vi "registrationEtlZDynamic.vi"() -> ()   [LabVIEW 2017]
uses:
  globalDevices.vi
  globalUtilities.vi
panel:
  in  "stop":bool
  out "z-profile":cluster{dbl[], dbl[]}[](graph)
  in  "newVolume":bool
  # "1. Check that the peak does not move. This will check that\nyou have the right etlLatencyShift\n2. Check that when you set a value you get the correct position\nin the other lens' space."
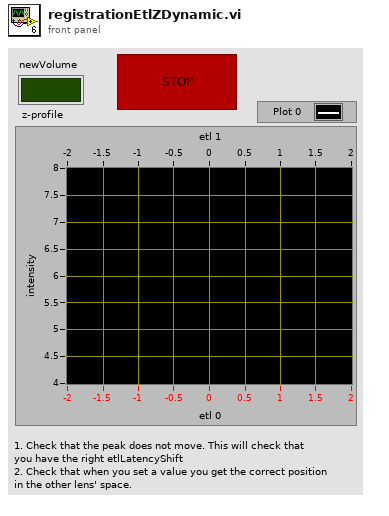
[diagram p1: front panel]
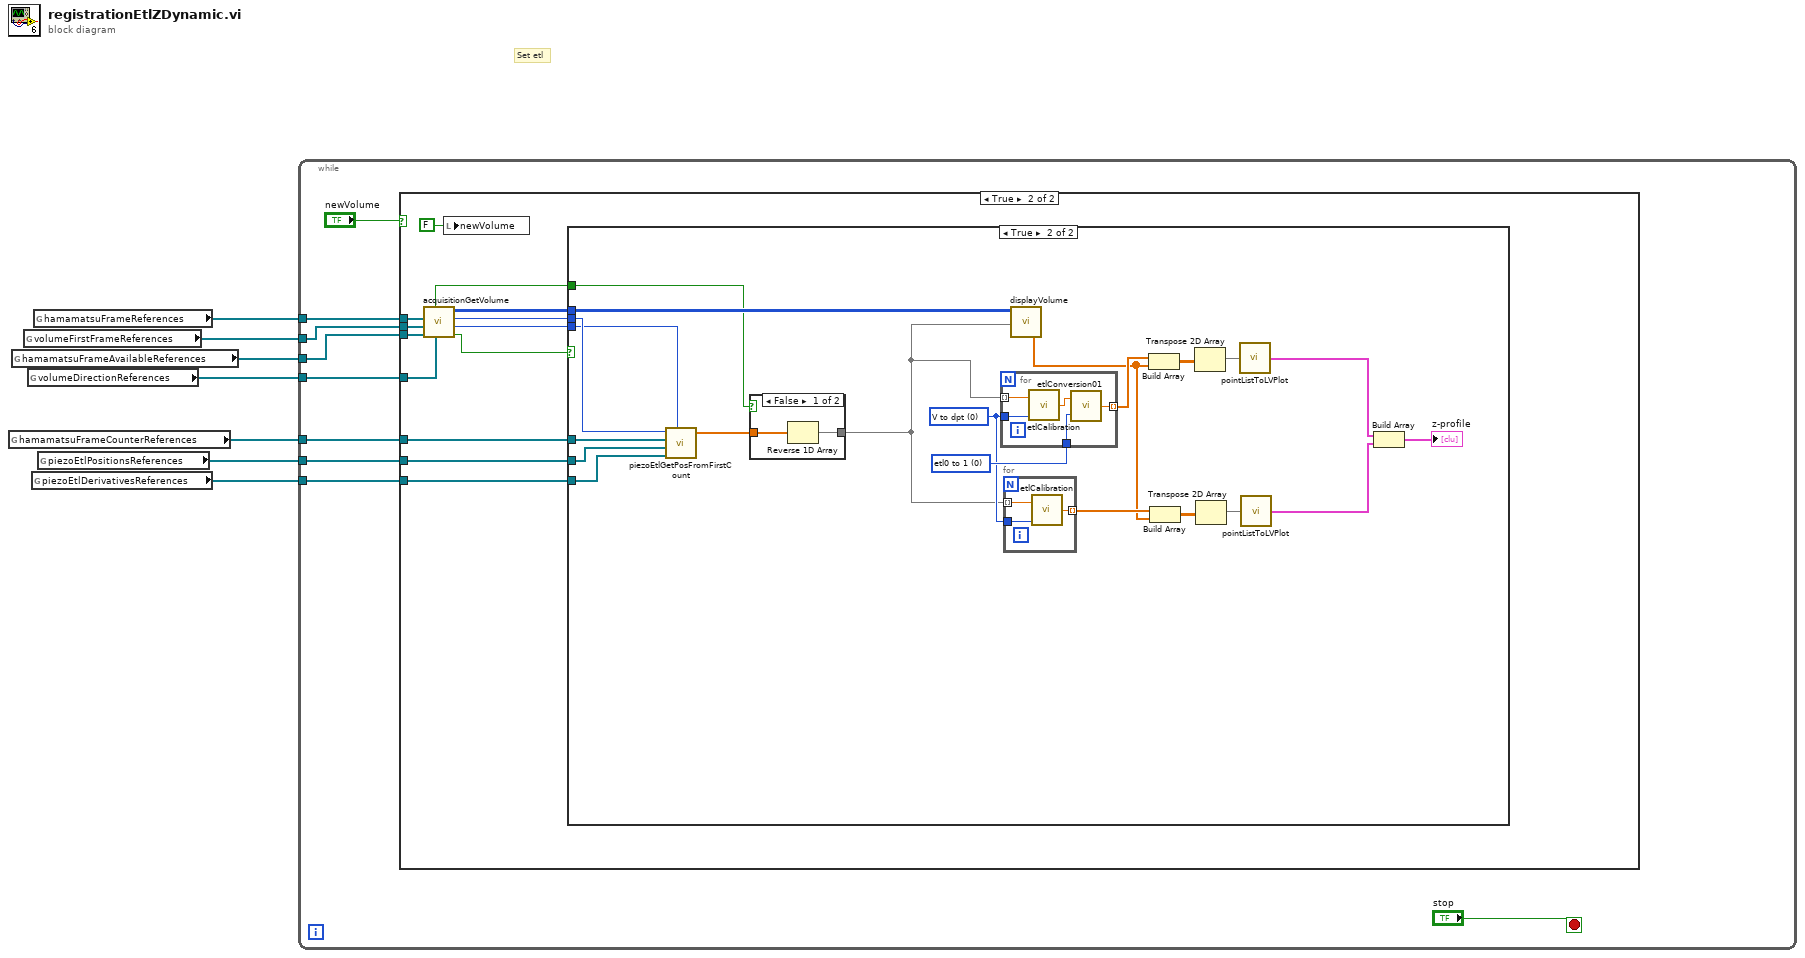
[diagram p0: block diagram]
diagram:
  # "Set etl"
  n1 = global read "globalDevices.vi" "hamamatsuFrameCounterReferences"() -> (w3:refnum<data-value>[])
  n2 = global read "globalDevices.vi" "hamamatsuFrameAvailableReferences"() -> (w5:refnum<data-value>[])
  n3 = global read "globalUtilities.vi" "volumeFirstFrameReferences"() -> (w6:refnum<data-value>[])
  n4 = global read "globalUtilities.vi" "volumeDirectionReferences"() -> (w4:refnum<data-value>[])
  n5 = global read "globalDevices.vi" "piezoEtlDerivativesReferences"() -> (w1:refnum<data-value>[])
  n6 = global read "globalDevices.vi" "hamamatsuFrameReferences"() -> (w7:refnum<data-value>[])
  n7 = global read "globalDevices.vi" "piezoEtlPositionsReferences"() -> (w2:refnum<data-value>[])
  n8 = while {
    tunnel: w7 -> [w16]
    tunnel: w6 -> [w15]
    tunnel: w5 -> [w14]
    tunnel: w4 -> [w13]
    tunnel: w3 -> [w12]
    tunnel: w2 -> [w11]
    tunnel: w1 -> [w10]
    stop <- "stop" stop-if-true
    n9 = case shown="True" "newVolume" {
      tunnel: w16 -> [_ w29]
      tunnel: w15 -> [_ w28]
      tunnel: w14 -> [_ w27]
      tunnel: w13 -> [_ w26]
      tunnel: w12 -> [_ w21]
      tunnel: w11 -> [_ w20]
      tunnel: w10 -> [_ w19]
      frame False {
      }
      frame True {
        n10 = call "acquisitionGetVolume.vi"("volumeDirectionReferences"=w26, "hamamatsuFrameAvailableReferences"=w27, "volumeFirstFrameReferences"=w28, "hamamatsuFrameReferences"=w29) -> ("success"=w25:bool, "numberOfFrames"=w22:u32, "absoluteCountFirstFrame"=w23:u32, "volume out"=w24:u16[][][], "volume direction out"=w17:bool)  [unwired: 1 in]
        n11 = local write "newVolume"(FALSE ("newVolume")) -> ()
        n12 = case shown="True" w25 {
          tunnel: w24 -> [_ w45]
          tunnel: w23 -> [_ w47]
          tunnel: w22 -> [_ w46]
          tunnel: w21 -> [_ w50]
          tunnel: w20 -> [_ w49]
          tunnel: w19 -> [_ w48]
          tunnel: w17 -> [_ w30]
          frame False {
          }
          frame True {
            w42 = u16 0 items=["etl0 to 1", "etl1 to 0"] ("mode")
            w40 = u16 0 items=["V to dpt", "dpt to V"] ("mode")
            n13 = call "piezoEtlGetPosFromFirstCount.vi"("firstFrameCount"=w47, "hamamatsuFrameCounterReferences"=w50, "piezoEtlPositionsReferences"=w49, "piezoEtlDerivativesReferences"=w48, "nFrames"=w46) -> ("piezoEtlPositions"=w32:dbl[])  [unwired: 2 out]
            n14 = case shown="False" w30 {
              tunnel: w32 -> [w52 w53]
              tunnel: [w51 w53] -> w31
              frame False {
                n15 = Reverse 1D Array(array=w52) -> (reversed array=w51:dbl[])
              }
              frame True {
              }
            }
            n16 = for {
              tunnel: w31 -> [w61] mode=indexing
              tunnel: w40 -> [w60]
              tunnel: w42 -> [w59]
              tunnel: [w57] -> w41 mode=indexing
              n17 = call "etlCalibration.vi"("mode"=w60, "in"=w61) -> ("out"=w58:dbl)
              n18 = call "etlConversion01.vi"("mode"=w59, "in"=w58) -> ("out"=w57:dbl)
            }
            n19 = for {
              tunnel: w31 -> [w56] mode=indexing
              tunnel: w40 -> [w55]
              tunnel: [w54] -> w37 mode=indexing
              n20 = call "etlCalibration.vi"("mode"=w55, "in"=w56) -> ("out"=w54:dbl)
            }
            n21 = call "displayVolume.vi"("frames"=w45, "z"=w31) -> ("z profile"=w36:dbl[])  [unwired: 12 in, 5 out]
            n22 = Build Array(w41, w36) -> (w44:dbl[][])
            n23 = Build Array(w37, w36) -> (w38:dbl[][])
            n24 = Transpose 2D Array(2D array=w44) -> (transposed array=w43:dbl[][])
            n25 = Transpose 2D Array(2D array=w38) -> (transposed array=w39:dbl[][])
            n26 = call "pointListToLVPlot.vi"("XY[N,d]"=w43) -> ("LV plot"=w35:cluster{dbl[], dbl[]})
            n27 = call "pointListToLVPlot.vi"("XY[N,d]"=w39) -> ("LV plot"=w34:cluster{dbl[], dbl[]})
            n28 = Build Array(w35, w34) -> (→"z-profile":cluster{dbl[], dbl[]}[])
          }
        }
      }
    }
  }
